vi "Construct Country.vi"(5 "Country in":refnum<class "Country.lvclass">, 8 "error in (no error)":errorcluster, 10 "Cities":refnum<class "City.lvclass">[](array[class]), 11 "Name":string) -> (0 "error out":errorcluster, 3 "Country":refnum<class "Country.lvclass">)   [LabVIEW 2017, in "Generic Object Serializer Tests.lvlib" / "Country.lvclass"]
uses:
  Country.lvclass
  City/City.lvclass
  Country.lvclass/Country.ctl
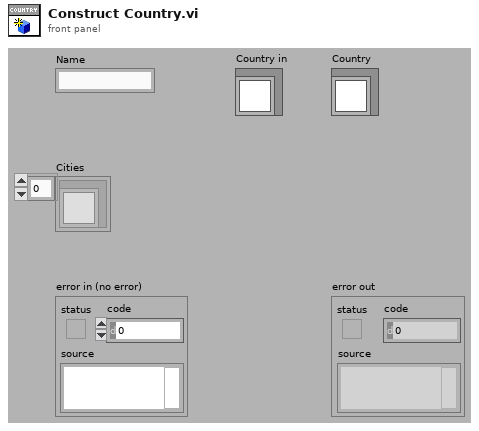
[diagram p1: front panel]
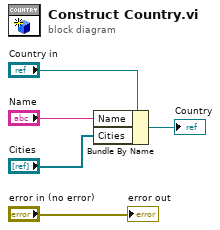
[diagram p0: block diagram]
diagram:
  n1 = Bundle By Name(cluster="Country in", "Name"="Name", "Cities"="Cities") -> (→"Country":refnum<class "Country.lvclass">)
  "error out" <- "error in (no error)"
